vi "Main.vi"() -> ()   [LabVIEW 2020]
doc: "Machine d'état simple"
uses:
  _Controls/Ctrl_states.ctl
  _Controls/Ctrl_local.ctl
panel:
  out "Display":cluster{"Num":dbl, "Char":string}
  in  "Pad":T1
  in  "Btn_Stop":bool
  in  "Btn_Error":bool
  out "error out":errorcluster caption="sortie d'erreur"
  in  "error in":errorcluster caption="entrée d'erreur"
  # "Calculatrice"
  # "Error command"
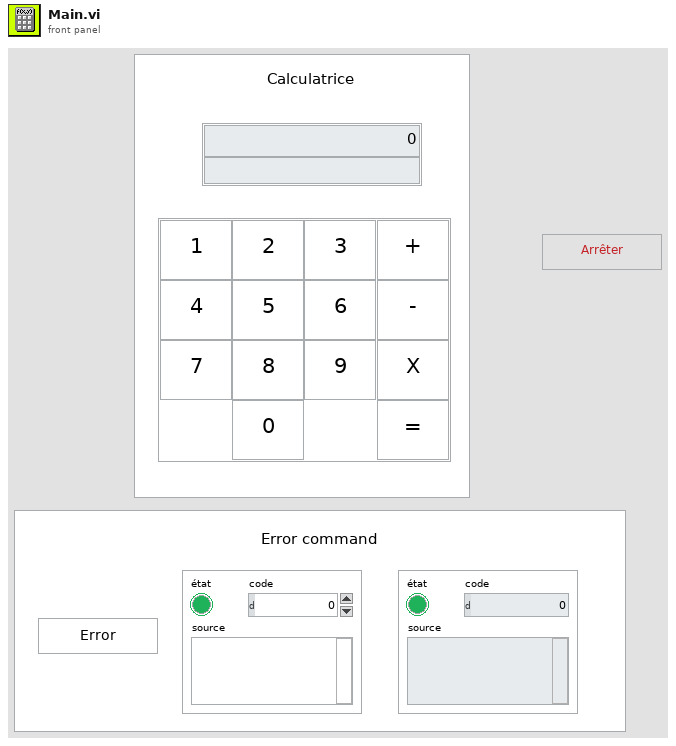
[diagram p1: front panel]
types:
  T1 = cluster{"Btn_1":bool, "Btn_2":bool, "Btn_3":bool, "Btn_4":bool, "Btn_5":bool, "Btn_6":bool, "Btn_7":bool, "Btn_8":bool, "Btn_9":bool, "Btn_0":bool, "Btn_+":bool, "Btn_-":bool, "Btn_X":bool, "Btn_=":bool}
  T2 = typedef "Ctrl_states.ctl" = enum16{"Initialisation", "Idle", "Stop", "Error", "Display", "Etat 1", "Etat 2", "Etat 3", "Btn_num", "Btn_operator"}
  T3 = typedef "Ctrl_local.ctl" = cluster{"State":T2, "Intermediaire":string, "Display":cluster{"Num":dbl, "Char":string}, "btn_char":string}
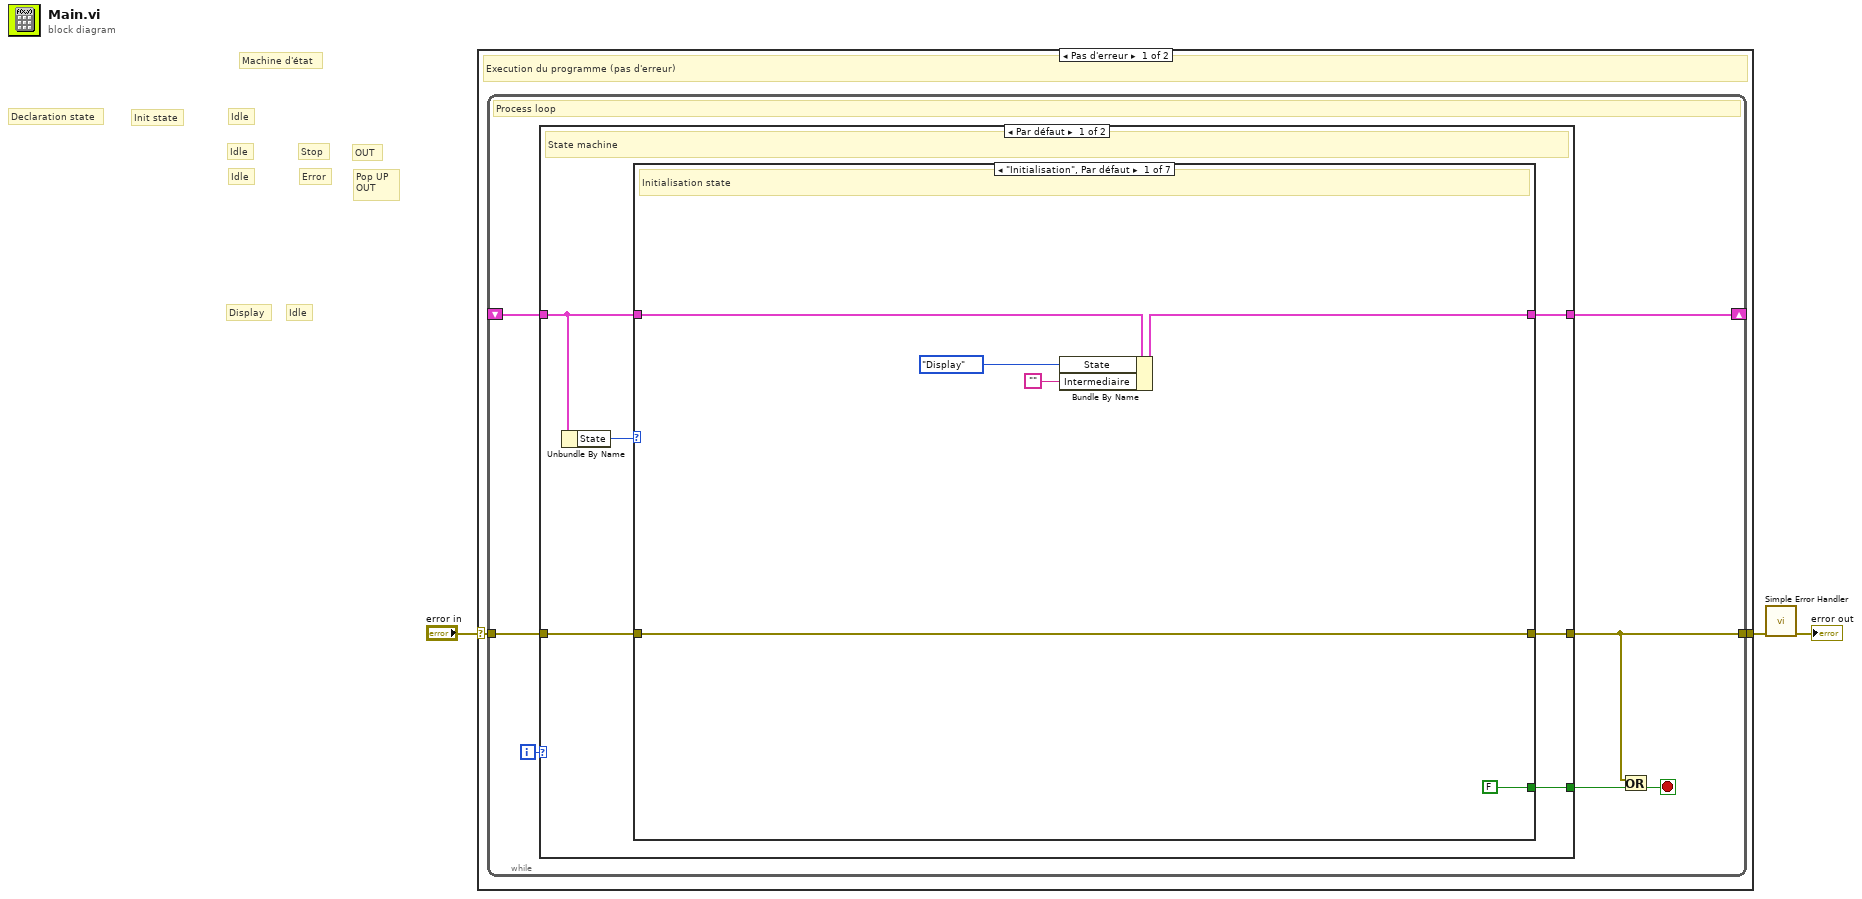
[diagram p0: block diagram]
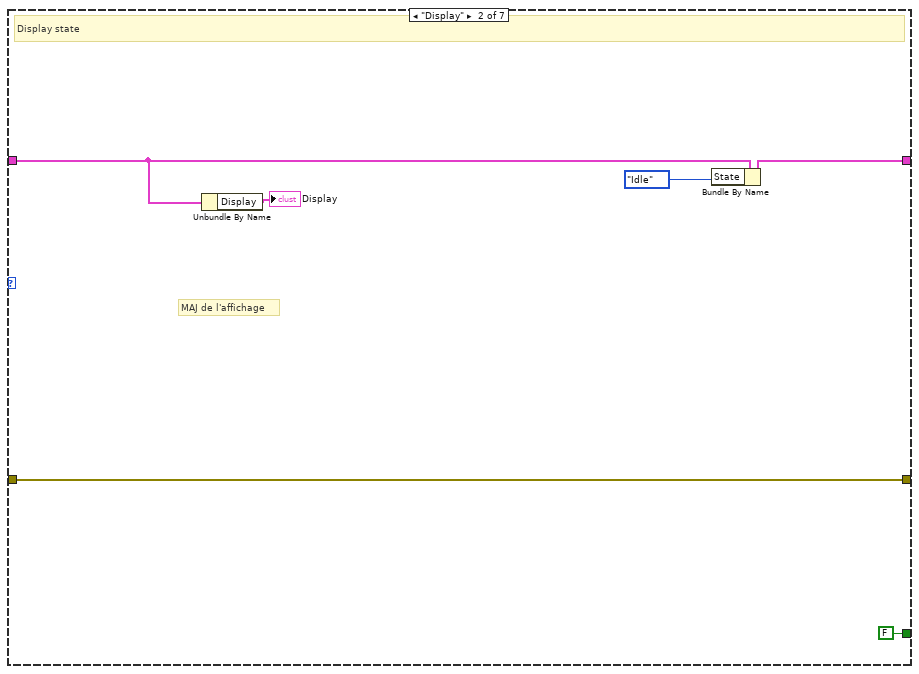
[diagram p2: hidden frame]
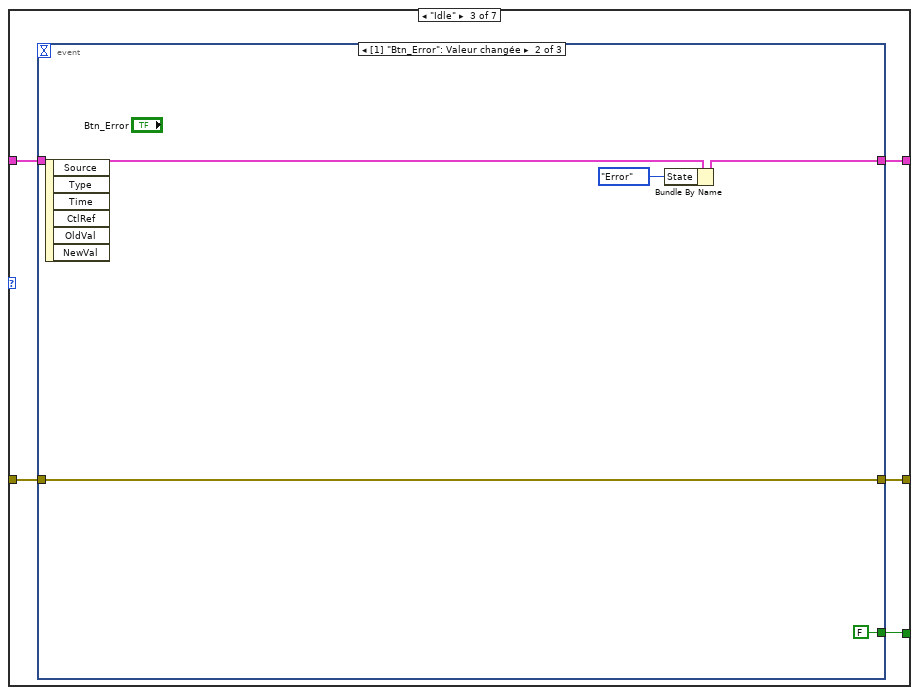
[diagram p3: hidden frame]
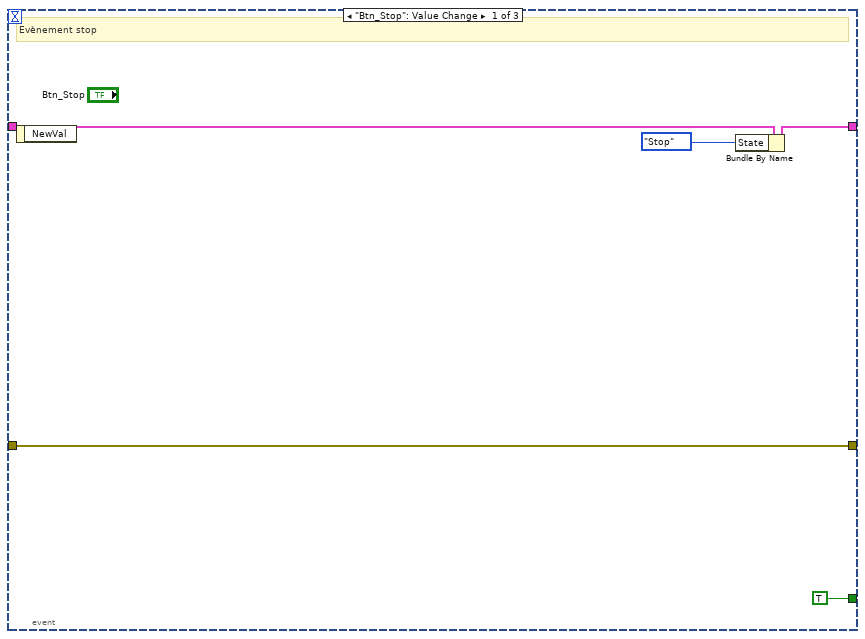
[diagram p4: hidden frame]
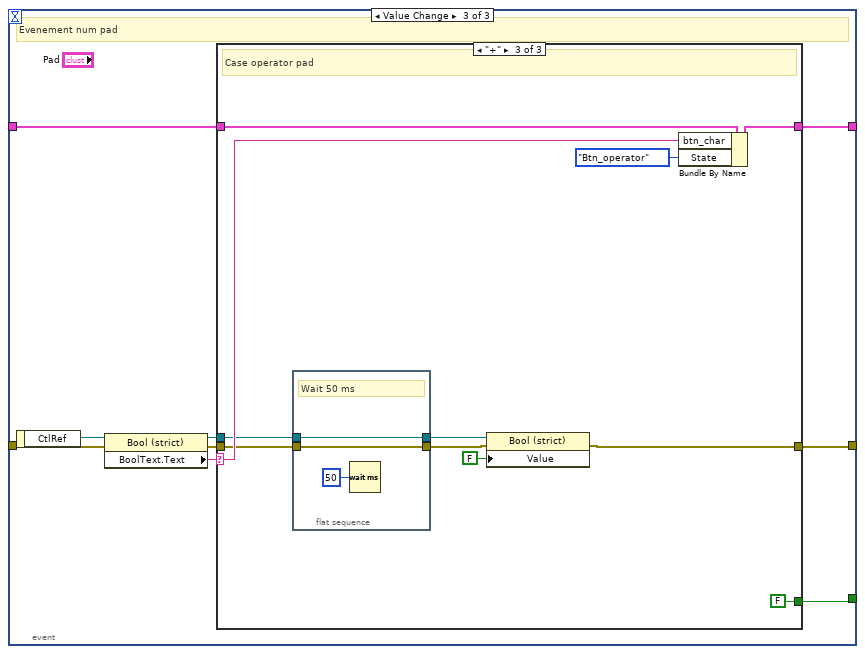
[diagram p5: hidden frame]
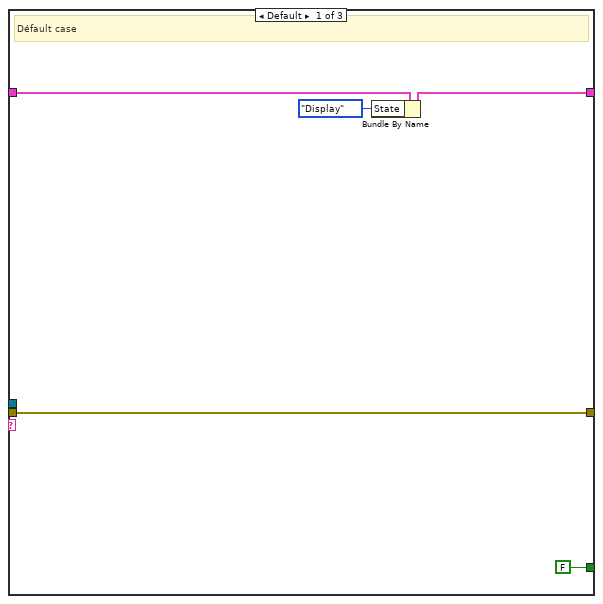
[diagram p6: hidden frame]
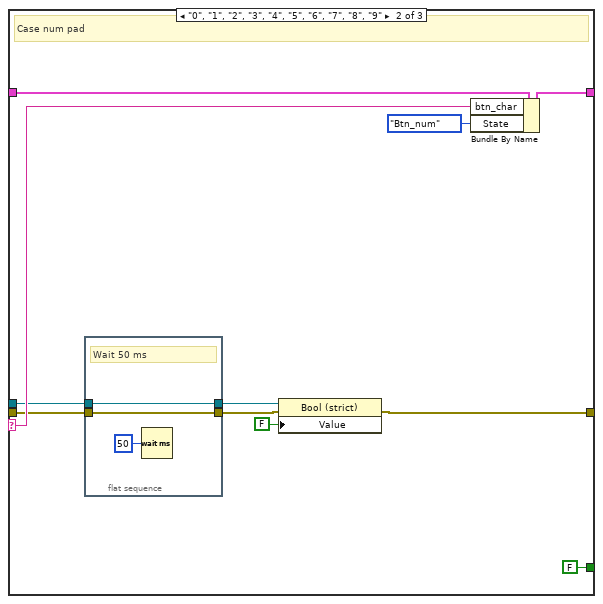
[diagram p7: hidden frame]
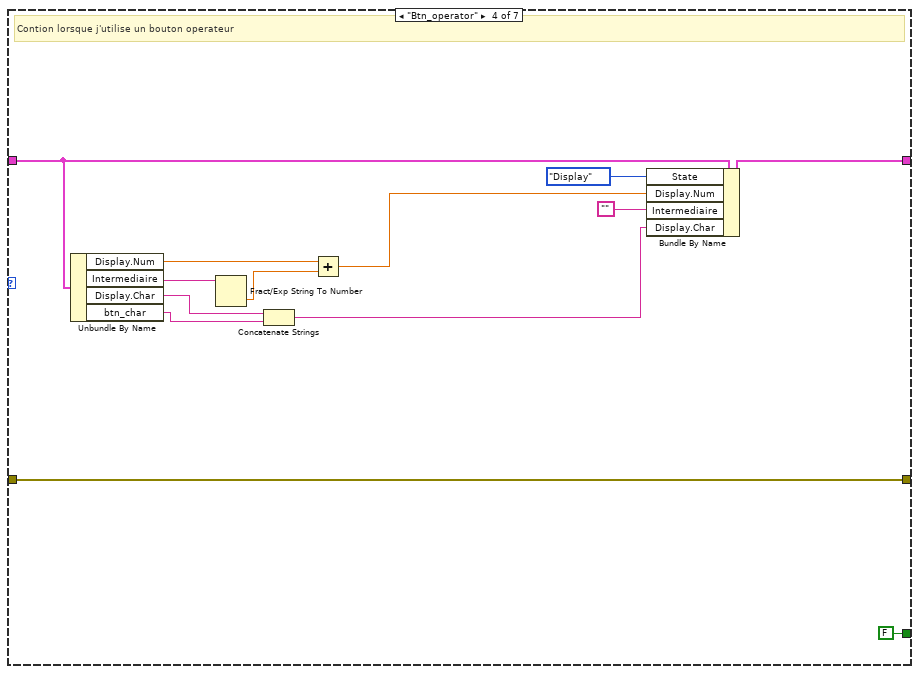
[diagram p8: hidden frame]
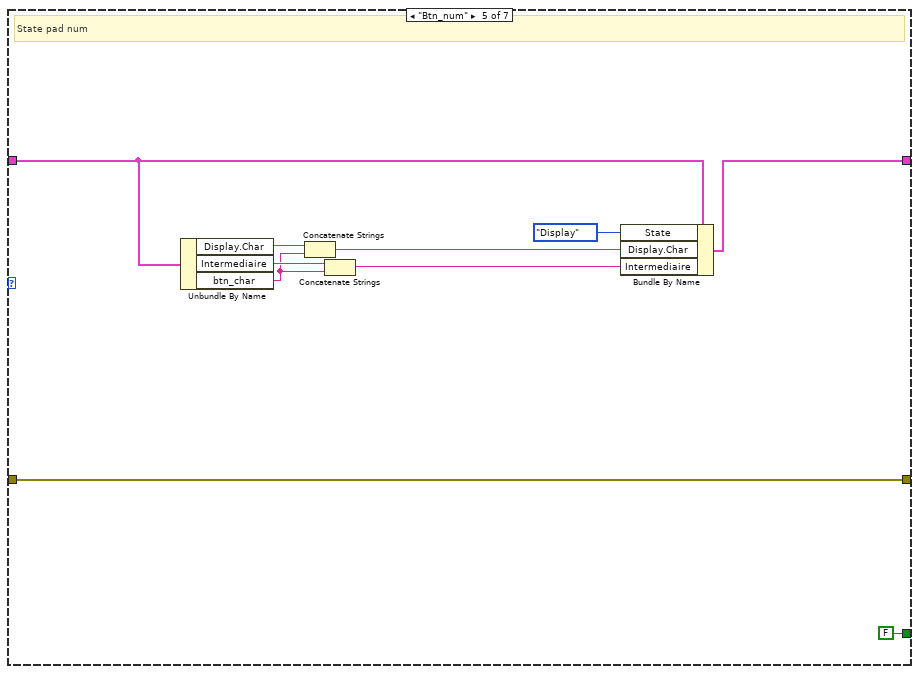
[diagram p9: hidden frame]
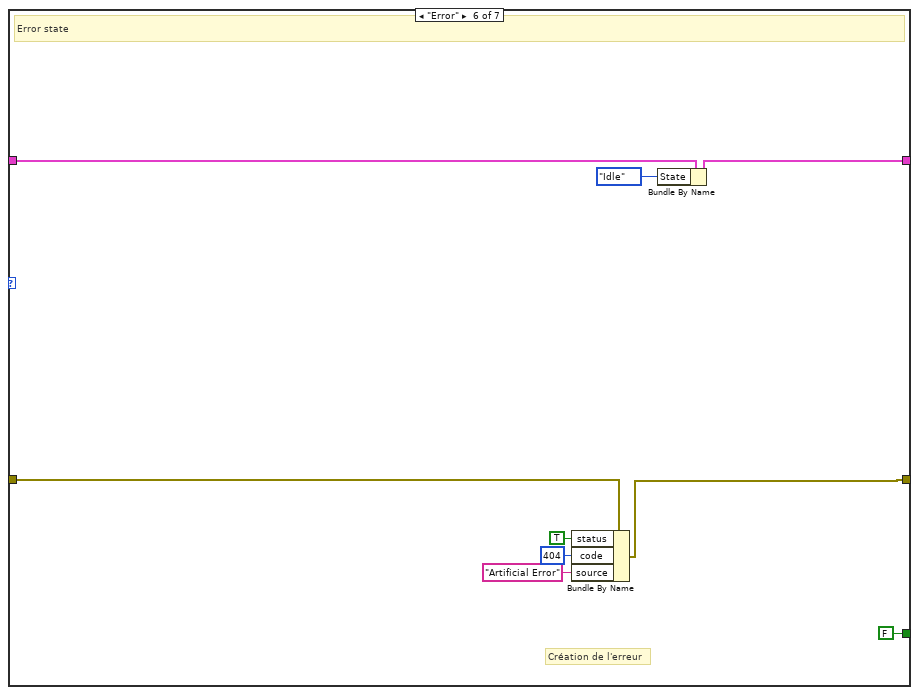
[diagram p10: hidden frame]
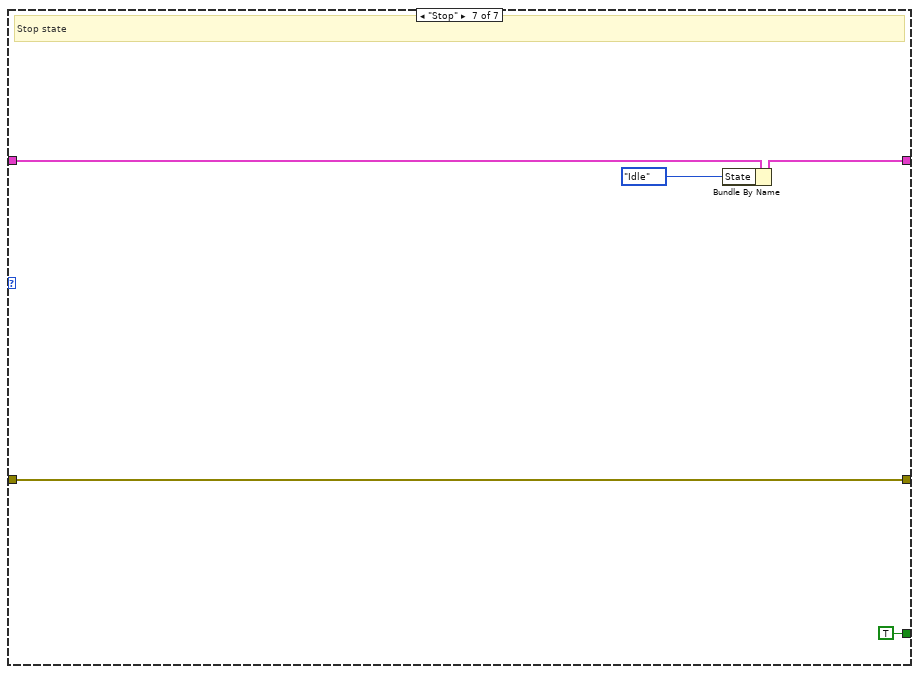
[diagram p11: hidden frame]
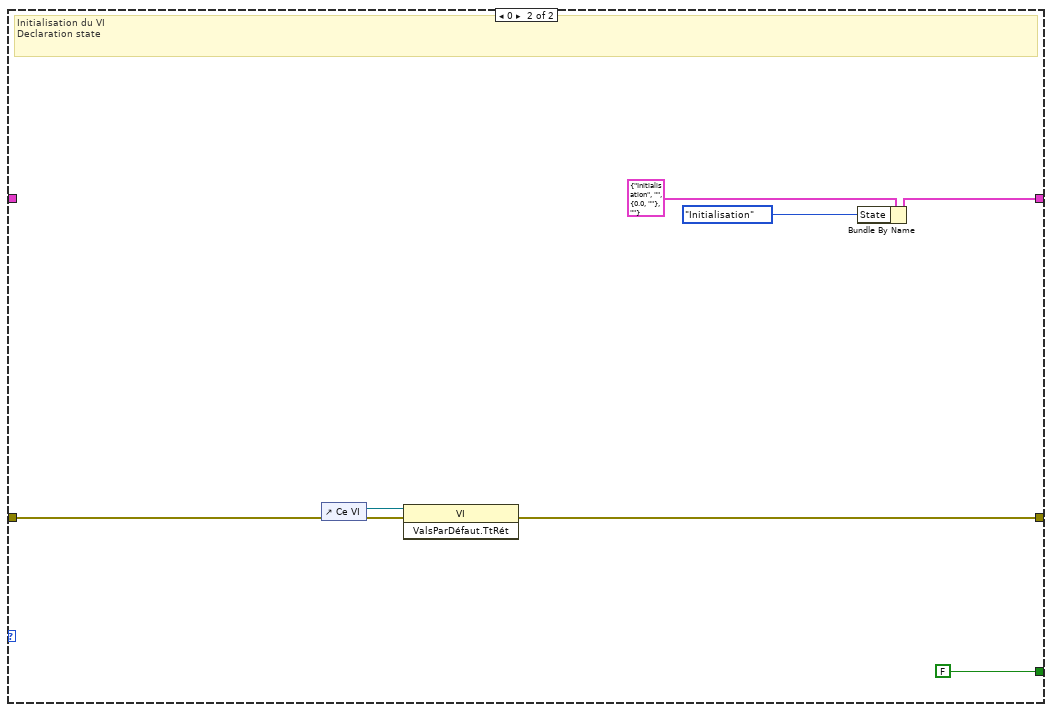
[diagram p12: hidden frame]
diagram:
  # "Idle"
  # "Display"
  # "Pop UP \nOUT"
  # "Error"
  # "Idle"
  # "OUT"
  # "Stop"
  # "Idle"
  # "Idle"
  # "Init state"
  # "Declaration state"
  # "Machine d'état"
  n1 = case shown="Pas d'erreur" "error in" {
    selector: "error in" -> [w5 w132]
    tunnel: [w4 w132] -> w2
    frame No Error {
      # "Execution du programme (pas d'erreur)"
      n2 = while {
        tunnel: w5 -> [w12]
        tunnel: [w8] -> w4
        shift-right: [w6] -> _
        shift-left: _ -> [w7]
        i -> [w11]
        stop <- w9 stop-if-true
        # "Process loop"
        n3 = case shown="Par défaut" w11 {
          tunnel: w12 -> [w18 w130]
          tunnel: [w16 w129] -> w8
          tunnel: [w17 FALSE] -> w10
          tunnel: [w15 w126] -> w6
          tunnel: w7 -> [w14 _]
          frame Default {
            # "State machine"
            n4 = Unbundle By Name(w14) -> ("State"=w13:T2)
            n5 = case shown="\"Initialisation\", Par défaut" w13 {
              tunnel: w18 -> [w23 w29 w35 w100 w110 w118 w124]
              tunnel: [FALSE FALSE w34 FALSE FALSE FALSE TRUE] -> w17
              tunnel: [w23 w29 w33 w100 w110 w117 w124] -> w16
              tunnel: w14 -> [w22 w30 w32 w97 w103 w113 w122]
              tunnel: [w21 w27 w31 w99 w102 w112 w121] -> w15
              frame "Initialisation", Default {
                # "Initialisation state"
                n6 = Bundle By Name(cluster=w22, "State"=Ctrl_states."Display", "Intermediaire"="") -> (w21:T3)
              }
              frame "Display" {
                # "MAJ de l'affichage"
                # "Display state"
                n7 = Unbundle By Name(w30) -> ("Display"=→"Display":cluster{"Num":dbl, "Char":string})
                n8 = Bundle By Name(cluster=w30, "State"=Ctrl_states."Idle") -> (w27:T3)
              }
              frame "Idle" {
                n9 = event shown="[1] \"Btn_Error\": Valeur changée" {
                  selector: _ -> [_ _ _]
                  dyn-events: _ -> [_ _ _]
                  timeout: _ -> [_ _ _]
                  tunnel: w35 -> [w39 w45 w53]
                  tunnel: [TRUE FALSE w49] -> w34
                  tunnel: [w39 w45 w50] -> w33
                  tunnel: w32 -> [w38 w43 w48]
                  tunnel: [w37 w42 w47] -> w31
                  event "Btn_Stop": Value Change {
                    # "Evènement stop"
                    n10 = event-data() -> ()  [unwired: 1 in, 1 out]
                    n11 = Bundle By Name(cluster=w38, "State"=Ctrl_states."Stop") -> (w37:T3)
                  }
                  event "Btn_Error": Value Change {
                    n12 = event-data() -> ()  [unwired: 1 in, 6 out]
                    n13 = Bundle By Name(cluster=w43, "State"=Ctrl_states."Error") -> (w42:T3)
                  }
                  event "Pad.Btn_1", "Pad.Btn_2", "Pad.Btn_3", "Pad.Btn_4", "Pad.Btn_5", "Pad.Btn_6", "Pad.Btn_7", "Pad.Btn_8", "Pad.Btn_9", "Pad.Btn_0", "Pad.Btn_+": Value Change {
                    # "Evenement num pad"
                    n14 = event-data() -> ("CtlRef"=w54:refnum<vi>)  [unwired: 1 in]
                    n15 = property class="Bool (strict)"(reference=w54, error in=w53) -> (reference out=w46:refnum<vi>, error out=w51:errorcluster, "BoolText.Text"=w52:string)
                    n16 = case shown="\"+\"" w52 {
                      selector: w52 -> [_ w67 w81]
                      tunnel: w51 -> [w59 w65 w79]
                      tunnel: [w59 w63 w77] -> w50
                      tunnel: [FALSE FALSE FALSE] -> w49
                      tunnel: w48 -> [w57 w69 w83]
                      tunnel: [w56 w68 w82] -> w47
                      tunnel: w46 -> [_ w62 w76]
                      frame Default {
                        # "Défault case"
                        n17 = Bundle By Name(cluster=w57, "State"=Ctrl_states."Display") -> (w56:T3)
                      }
                      frame "0", "1", "2", "3", "4", "5", "6", "7", "8", "9" {
                        # "Case num pad"
                        n18 = flat-sequence {
                          tunnel: w65 -> [w73]
                          tunnel: [w73] -> w64
                          tunnel: w62 -> [w72]
                          tunnel: [w72] -> w61
                          frame #0 {
                            # "Wait 50 ms"
                            n19 = Wait (ms)(milliseconds to wait=u32 50 ("attente (ms)")) -> ()  [unwired: 1 out]
                          }
                        }
                        n20 = property class="Bool (strict)"(reference=w61, error in=w64, "Value"=FALSE ("Valeur")) -> (error out=w63:errorcluster)  [unwired: 1 out]
                        n21 = Bundle By Name(cluster=w69, "btn_char"=w67, "State"=Ctrl_states."Btn_num") -> (w68:T3)
                      }
                      frame "+" {
                        # "Case operator pad"
                        n22 = flat-sequence {
                          tunnel: w79 -> [w87]
                          tunnel: [w87] -> w78
                          tunnel: w76 -> [w86]
                          tunnel: [w86] -> w75
                          frame #0 {
                            # "Wait 50 ms"
                            n23 = Wait (ms)(milliseconds to wait=u32 50 ("attente (ms)")) -> ()  [unwired: 1 out]
                          }
                        }
                        n24 = property class="Bool (strict)"(reference=w75, error in=w78, "Value"=FALSE ("Valeur")) -> (error out=w77:errorcluster)  [unwired: 1 out]
                        n25 = Bundle By Name(cluster=w83, "btn_char"=w81, "State"=Ctrl_states."Btn_operator") -> (w82:T3)
                      }
                    }
                  }
                }
              }
              frame "Btn_operator" {
                # "Contion lorsque j'utilise un bouton operateur"
                n26 = Unbundle By Name(w97) -> ("Display.Num"=w95:dbl, "Intermediaire"=w96:string, "Display.Char"=w92:string, "btn_char"=w91:string)
                n27 = Fract/Exp String To Number(string=w96) -> (number=w94:dbl)  [unwired: 3 in, 1 out]
                n28 = Concatenate Strings(w92, w91) -> (w90:string)
                n29 = Add(x=w95, y=w94) -> (x+y=w93:dbl)
                n30 = Bundle By Name(cluster=w97, "State"=Ctrl_states."Display", "Display.Num"=w93, "Intermediaire"="", "Display.Char"=w90) -> (w99:T3)
              }
              frame "Btn_num" {
                # "State pad num"
                n31 = Unbundle By Name(w103) -> ("Display.Char"=w105:string, "Intermediaire"=w107:string, "btn_char"=w101:string)
                n32 = Concatenate Strings(w105, w101) -> (w106:string)
                n33 = Concatenate Strings(w107, w101) -> (w108:string)
                n34 = Bundle By Name(cluster=w103, "State"=Ctrl_states."Display", "Display.Char"=w106, "Intermediaire"=w108) -> (w102:T3)
              }
              frame "Error" {
                # "Création de l'erreur"
                # "Error state"
                n35 = Bundle By Name(cluster=w118, "status"=TRUE, "code"=404, "source"="Artificial Error") -> (w117:errorcluster)
                n36 = Bundle By Name(cluster=w113, "State"=Ctrl_states."Idle") -> (w112:T3)
              }
              frame "Stop" {
                # "Stop state"
                n37 = Bundle By Name(cluster=w122, "State"=Ctrl_states."Idle") -> (w121:T3)
              }
            }
          }
          frame 0 {
            # "Initialisation du VI\nDeclaration state"
            n38 = control-ref of="Ce VI"() -> (w131:refnum<vi>)
            n39 = invoke class="VI" method="ValsParDéfaut.TtRét"(reference=w131, error in=w130) -> (error out=w129:errorcluster)  [unwired: 1 in, 2 out]
            n40 = Bundle By Name(cluster=T3 {"State"=enum."Initialisation", "Intermediaire"="", "Display"={"Num"=0.0, "Char"=""}, "btn_char"=""} ("Local"), "State"=Ctrl_states."Initialisation") -> (w126:T3)
          }
        }
        n41 = Or(x=w8, y=w10) -> (x .or. y?=w9:bool)
      }
    }
    frame Error {
      # "non execution du programme (erreur)"
    }
  }
  n42 = call <vilib>:"Simple Error Handler.vi"("error in (no error)"=w2) -> ("error out"=→"error out":errorcluster)  [unwired: 4 in, 4 out]
